vi "Query ILC.vi"(8 "error in (no error)":errorcluster, 11 "Model in":refnum<class "Model.lvclass">) -> (0 "error out":errorcluster, 3 "Model out":refnum<class "Model.lvclass">)   [LabVIEW 2015, in "Model.lvclass"]
uses:
  Model.lvclass
  Model.lvclass/Model.ctl
  Common_RT_Modbus/DynamicFrameParser/DynamicFrameParser.lvclass
  Modbus/DesktopModbus/DesktopModbus.lvclass
  Common_RT_FAILC/FAILC/FAILC.lvclass
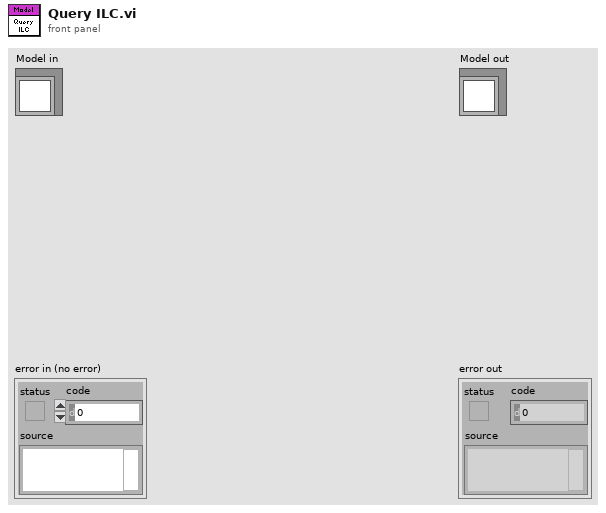
[diagram p1: front panel]
types:
  T1 = typedef "RTModbus.lvlib/Frame.ctl" = cluster{"Data":u8[], "WaitForTrigger":bool, "WaitForRx":u16, "TriggerIRQ":bool, "DelayTicks":u16, "DelayMicroseconds":u16, "DelayMilliseconds":u16}
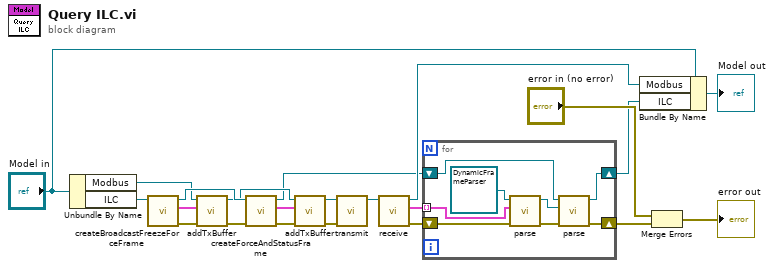
[diagram p0: block diagram]
diagram:
  n1 = Unbundle By Name("Model in") -> ("Modbus"=w20:refnum<class "DesktopModbus.lvclass">, "ILC"=w22:refnum<class "FAILC.lvclass">)
  n2 = call "createBroadcastFreezeForceFrame.vi"("FAILC in"=w22) -> ("error out"=w16:errorcluster, "Frame"=w18:T1, "FAILC out"=w21:refnum<class "FAILC.lvclass">)  [unwired: 8 in]
  n3 = call-dynamic "addTxBuffer.vi"("error in (no error)"=w16, "Frame"=w18, "DesktopModbus in"=w20) -> ("error out"=w15:errorcluster, "DesktopModbus out"=w19:refnum<class "DesktopModbus.lvclass">)  [unwired: 7 in]
  n4 = call "createForceAndStatusFrame.vi"("error in (no error)"=w15, "FAILC in"=w21) -> ("error out"=w14:errorcluster, "Frame"=w17:T1, "FAILC out"=w5:refnum<class "FAILC.lvclass">)  [unwired: 7 in]
  n5 = call-dynamic "addTxBuffer.vi"("error in (no error)"=w14, "Frame"=w17, "DesktopModbus in"=w19) -> ("error out"=w12:errorcluster, "DesktopModbus out"=w13:refnum<class "DesktopModbus.lvclass">)  [unwired: 7 in]
  n6 = call-dynamic "transmit.vi"("error in (no error)"=w12, "DesktopModbus in"=w13) -> ("DesktopModbus out"=w7:refnum<class "DesktopModbus.lvclass">)  [unwired: 8 in, 1 out]
  n7 = call-dynamic "receive.vi"("DesktopModbus in"=w7) -> ("error out"=w3:errorcluster, "Data"=w4:T1[], "DesktopModbus out"=w6:refnum<class "DesktopModbus.lvclass">)  [unwired: 8 in]
  n8 = for {
    tunnel: w4 -> [w29] mode=indexing
    shift-right: [w26] -> w2
    shift-left: w5 -> [w28]
    shift-right: [w24] -> w1
    shift-left: w3 -> [w23]
    n9 = call "parse.vi"("error in (no error)"=w23, "Frame"=w29, "FrameParser in"=refnum<class "DynamicFrameParser.lvclass"> refnum ("RTModbus.lvlib:DynamicFrameParser.lvclass")) -> ("error out"=w25:errorcluster, "FrameParser out"=w27:refnum<class "DynamicFrameParser.lvclass">)  [unwired: 7 in]
    n10 = call-dynamic "parse.vi"("error in (no error)"=w25, "DynamicFrameParser"=w27, "FAILC in"=w28) -> ("error out"=w24:errorcluster, "FAILC out"=w26:refnum<class "FAILC.lvclass">)  [unwired: 6 in, 1 out]
  }
  n11 = Bundle By Name(cluster="Model in", "Modbus"=w6, "ILC"=w2) -> (→"Model out":refnum<class "Model.lvclass">)
  n12 = Merge Errors("error in (no error)", w1) -> (→"error out":errorcluster)
